vi "Extract Waveform Data.vi"(0 "Next Sample Start Position":i32, 5 "Previous Amplitudes":dbl[](array[numeric]), 9 "data":waveform(dbl)[](array[waveform]), 11 "error in":errorcluster) -> (4 "Next Sample Start Position":i32, 6 "Current Max":dbl, 8 "Levels":dbl[](array[numeric]), 15 "error out":errorcluster)   [LabVIEW 2015, in "LabVIEW Interface for Arduino.lvlib"]
uses:
  <vilib>/LabVIEW Interface for Arduino/LabVIEW Interface for Arduino.lvlib
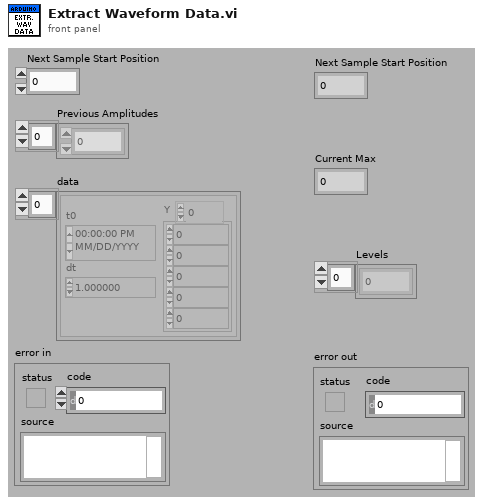
[diagram p1: front panel]
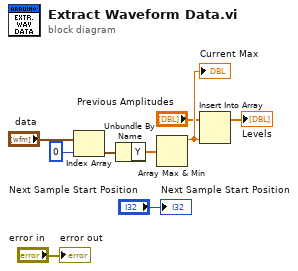
[diagram p0: block diagram]
diagram:
  n1 = Index Array(array="data", index=0) -> (element=w6:waveform(dbl))
  n2 = Unbundle By Name(w6) -> ("Y"=w8:dbl[])
  n3 = Array Max & Min(array=w8) -> (max value=w9:dbl)  [unwired: 3 out]
  "Current Max" <- w9
  n4 = Insert Into Array(array="Previous Amplitudes", new element=w9) -> (→"Levels":dbl[])  [unwired: 1 in]
  "error out" <- "error in"
  "Next Sample Start Position" <- "Next Sample Start Position"
